vi "Get Parent Directory.vi"(8 "error in (no error)":errorcluster caption="错误输入（无错误）", 10 "路径":path) -> (0 "error out":errorcluster caption="错误输出")   [LabVIEW 2012, in "Directory.lvclass"]
uses:
  Directory.lvclass
panel:
  out "GetParent":refnum<k24>
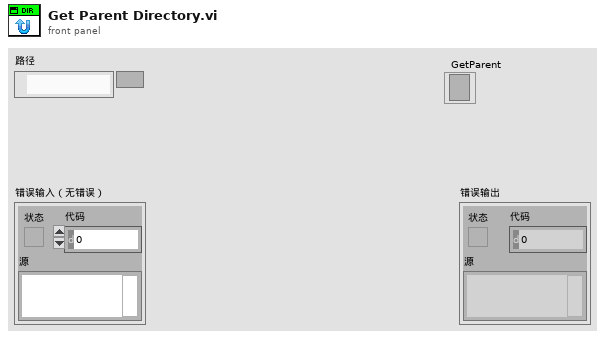
[diagram p1: front panel]
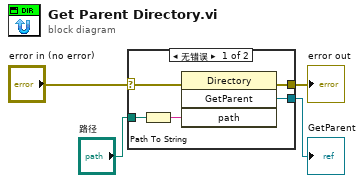
[diagram p0: block diagram]
diagram:
  n1 = case shown="无错误" "error in (no error)" {
    selector: "error in (no error)" -> [w9 w10]
    tunnel: [w8 w10] -> w3
    tunnel: "路径" -> [w7 _]
    tunnel: [w5 _] -> w1
    frame No Error {
      n2 = Path To String(path=w7) -> (string=w6:string)
      n3 = invoke on="调用节点" class="Directory" method="GetParent"(error in=w9, "path"=w6) -> (error out=w8:errorcluster, "GetParent"=w5:refnum<k24>)  [unwired: 2 in, 2 out]
    }
    frame Error {
    }
  }
  "error out" <- w3
  "GetParent" <- w1
